vi "Create Asserts Folder.vi"(8 "error in (no error)":errorcluster, 11 "Folder Path":path) -> (0 "error out":errorcluster)   [LabVIEW 2016]
doc: "Checks if a folder to store the assert vi's in exists already, if not it creates one in a sub-directory of the folder with vi quick drop was launched from in"
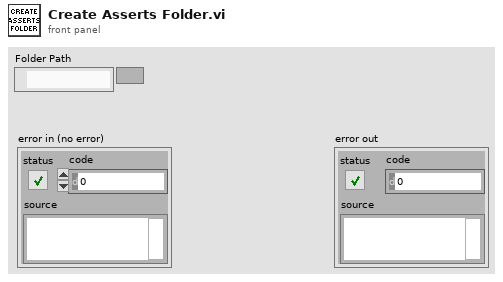
[diagram p1: front panel]
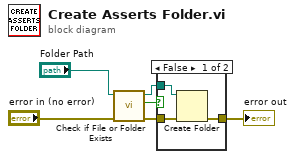
[diagram p0: block diagram]
diagram:
  n1 = call <vilib>:"Check if File or Folder Exists.vi"("error in (no error)"="error in (no error)", "path"="Folder Path") -> ("error out"=w1:errorcluster, "file or folder exists?"=w4:bool, "dup path"=w5:path)  [unwired: 7 in]
  n2 = case shown="False" w4 {
    tunnel: w1 -> [w9 w10]
    tunnel: [w8 w10] -> w3
    tunnel: w5 -> [w7 _]
    frame False {
      n3 = Create Folder(path (use dialog)=w7, error in=w9) -> (error out=w8:errorcluster)  [unwired: 1 in, 2 out]
    }
    frame True {
    }
  }
  "error out" <- w3
